vi "change_input.vi"(8 "error in":errorcluster, 9 "new vi path in":path, 10 "name or relative path in":string, 11 "new class path in":path) -> (0 "error out":errorcluster)   [LabVIEW 2010]
panel:
  out "number of replacements":i32
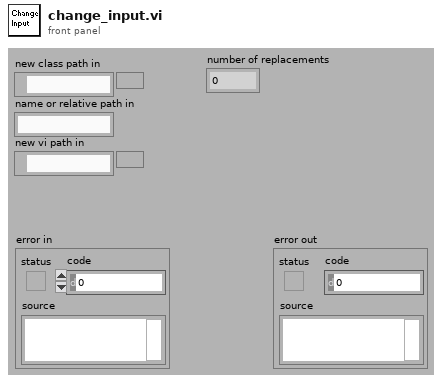
[diagram p1: front panel]
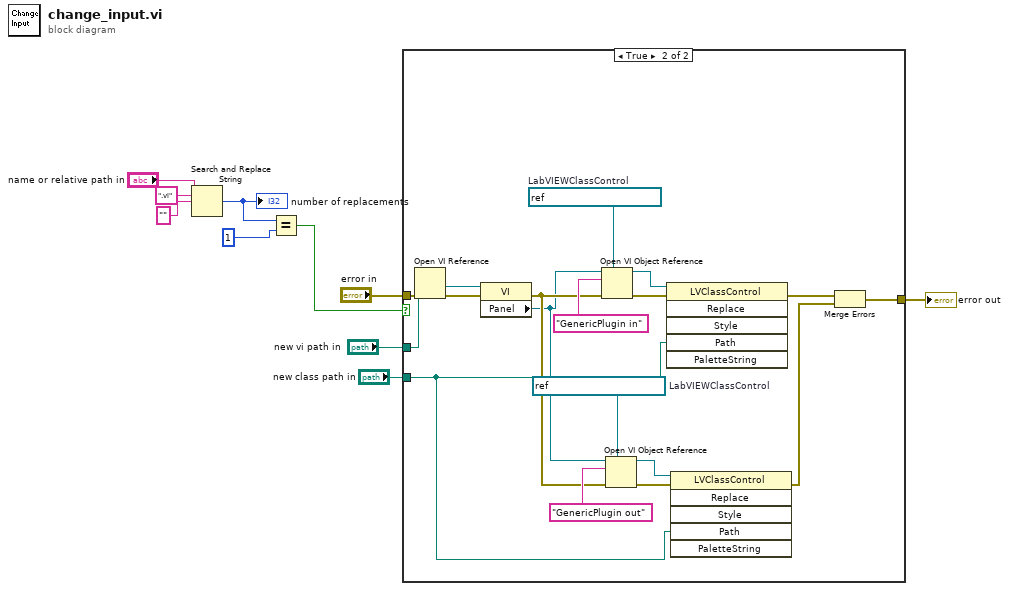
[diagram p0: block diagram]
diagram:
  n1 = Search and Replace String(input string="name or relative path in", search string=".vi", replace string="" ("replace string (\"\")")) -> (number of replacements=w6:i32)  [unwired: 5 in, 3 out]
  "number of replacements" <- w6
  n2 = Equal?(x=w6, y=1) -> (x = y?=w8:bool)
  n3 = case shown="True" w8 {
    tunnel: "error in" -> [w11 w25]
    tunnel: "new vi path in" -> [_ w23]
    tunnel: "new class path in" -> [_ w15]
    tunnel: [w11 w12] -> w7
    frame False {
    }
    frame True {
      w21 = refnum<vi> refnum  # LabVIEWClassControl
      w22 = refnum<vi> refnum  # LabVIEWClassControl
      n4 = Open VI Reference(vi path=w23, error in (no error)=w25) -> (vi reference=w27:refnum<vi>, error out=w24:errorcluster)  [unwired: 4 in]
      n5 = property class="VI"(reference=w27, error in=w24) -> (error out=w17:errorcluster, "Panel"=w16:refnum<vi>)  [unwired: 1 out]
      n6 = Open VI Object Reference(7:w22, 8:w17, 10:"GenericPlugin in" ("name/order"), 11:w16) -> (0:w26:errorcluster, 3:w29:refnum<vi>)
      n7 = Open VI Object Reference(7:w21, 8:w17, 10:"GenericPlugin out" ("name/order"), 11:w16) -> (0:w20:errorcluster, 3:w18:refnum<vi>)
      n8 = invoke class="LVClassControl" method="Replace"(reference=w29, error in=w26, "Path"=w15) -> (error out=w14:errorcluster)  [unwired: 3 in, 5 out]
      n9 = invoke class="LVClassControl" method="Replace"(reference=w18, error in=w20, "Path"=w15) -> (error out=w13:errorcluster)  [unwired: 3 in, 5 out]
      n10 = Merge Errors(w14, w13) -> (w12:errorcluster)
    }
  }
  "error out" <- w7
